vi "setChannel.vi"(8 "error in (no error)":errorcluster, 10 "Channel.lvclass":refnum<class "Channel.lvclass">, 11 "RfRamp.lvclass in":refnum<class "RfRamp.lvclass">) -> (0 "error out":errorcluster, 3 "RfRamp.lvclass out":refnum<class "RfRamp.lvclass">)   [LabVIEW 2009, in "Tools.lvlib" / "Scripting.lvlib" / "RfRamp.lvclass"]
uses:
  RfRamp.lvclass
  DatabaseHelpers/Database Objects/Channel/Channel.lvclass
  Rf Event/rf.lvclass
  RfRamp.lvclass/RfRamp.ctl
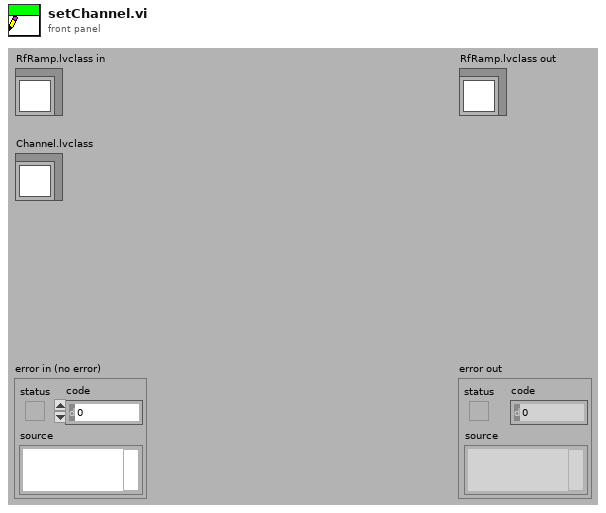
[diagram p1: front panel]
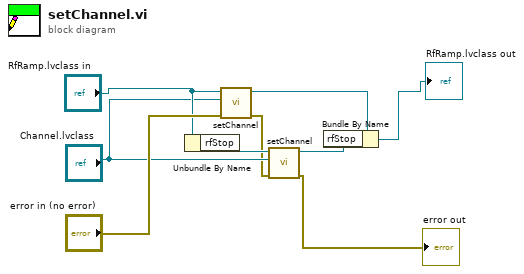
[diagram p0: block diagram]
diagram:
  n1 = Unbundle By Name("RfRamp.lvclass in") -> ("rfStop"=w7:refnum<class "rf.lvclass">)
  n2 = call-parent "setChannel.vi"("error in (no error)"="error in (no error)", "Channel.lvclass"="Channel.lvclass", "rf.lvclass in"="RfRamp.lvclass in") -> ("error out"=w1:errorcluster, "rf.lvclass out"=w5:refnum<class "RfRamp.lvclass">)  [unwired: 7 in]
  n3 = call-parent "setChannel.vi"("error in (no error)"=w1, "Channel.lvclass"="Channel.lvclass", "rf.lvclass in"=w7) -> ("error out"=→"error out":errorcluster, "rf.lvclass out"=w2:refnum<class "rf.lvclass">)  [unwired: 7 in]
  n4 = Bundle By Name(cluster=w5, "rfStop"=w2) -> (→"RfRamp.lvclass out":refnum<class "RfRamp.lvclass">)
